vi "Inspect Certificate.vi"(11 "Certificate string":string) -> (3 "Certificates":T1(array[cluster]))   [LabVIEW 2013, in "Certification Authority.lvclass"]
uses:
  Certification Authority.lvclass
  <vilib>/LabVIEW Open Source Project/OpenSerializer.Base64/Base64_CharSet.vi
  <vilib>/Utility/error.llb/Error Cluster From Error Code.vi
  <vilib>/regexp/Match Regular Expression.xnode
  <vilib>/LabVIEW Open Source Project/OpenSerializer.Base64/Serializer.Base64.lvclass
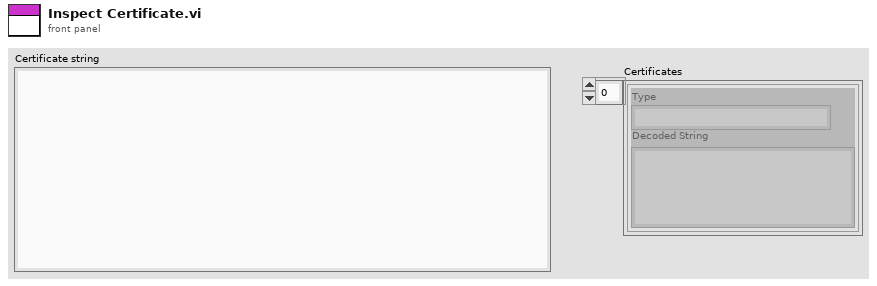
[diagram p1: front panel]
types:
  T1 = cluster{"Type":string, "Decoded String":string}[]
  T2 = cluster{"submatch 1":string, "spreadsheet string":string}
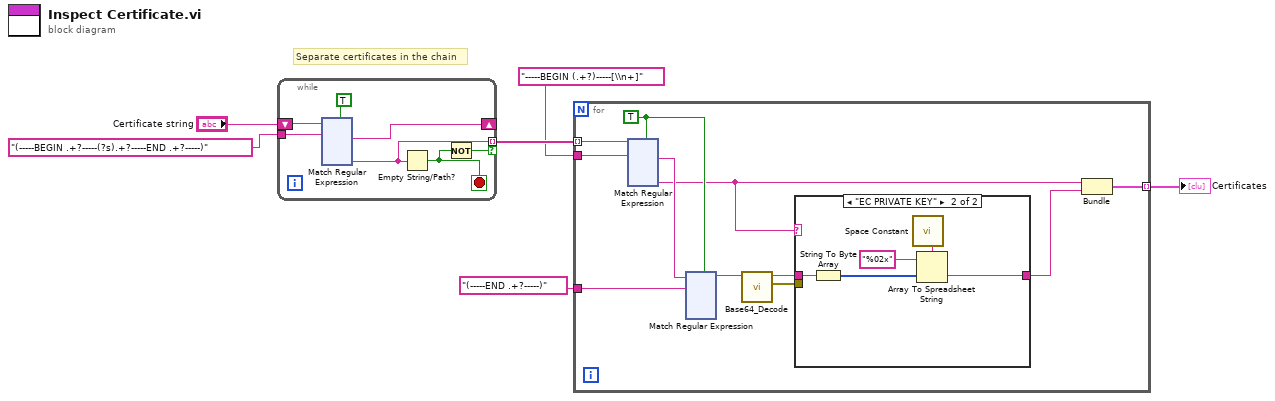
[diagram p0: block diagram]
diagram:
  # "Separate certificates in the chain"
  n1 = while {
    tunnel: "(-----BEGIN .+?-----(?s).+?-----END .+?-----)" ("regular expression") -> [w13]
    shift-right: [w11] -> _
    shift-left: "Certificate string" -> [w12]
    tunnel: [w9] -> w5 mode=indexing if=w8
    stop <- w7 stop-if-true
    n2 = xnode "Match Regular Expression"("input string"=w12, "regular expression"=w13, "multiline? (F)"=TRUE) -> ("after match"=w11:string, "submatch 1"=w9:string)  [unwired: 3 in, 4 out]
    n3 = Empty String/Path?(string/path=w9) -> (empty?=w7:bool)
    n4 = Not(x=w7) -> (.not. x?=w8:bool)
  }
  n5 = for {
    tunnel: w5 -> [w140] mode=indexing
    tunnel: "-----BEGIN (.+?)-----[\\n+]" ("regular expression") -> [w139]
    tunnel: "(-----END .+?-----)" ("regular expression") -> [w136]
    tunnel: [w134] -> w1 mode=indexing
    w137 = TRUE ("multiline? (F)")
    n6 = xnode "Match Regular Expression"("input string"=w140, "regular expression"=w139, "multiline? (F)"=w137) -> ("after match"=w138:string, "submatch 1"=w133:string)  [unwired: 3 in, 4 out]
    n7 = xnode "Match Regular Expression"("input string"=w138, "regular expression"=w136, "multiline? (F)"=w137) -> ("before match"=w135:string)  [unwired: 3 in, 5 out]
    n8 = call <vilib>:"Base64_Decode.vi"("Base64 String"=w135) -> ("error out"=w130:errorcluster, "Decoded String"=w132:string)  [unwired: 9 in]
    n9 = case shown="\"EC PRIVATE KEY\"" w133 {
      tunnel: w132 -> [w141 w146]
      tunnel: [w141 w145] -> w131
      tunnel: w130 -> [_ _]
      frame Default {
      }
      frame "EC PRIVATE KEY" {
        n10 = String To Byte Array(string=w146) -> (unsigned byte array=w144:u8[])
        n11 = call <vilib>:"Space Constant.vi"() -> ("String"=w142:string)
        n12 = Array To Spreadsheet String(delimiter (Tab)=w142, array=w144, 3:"%02x" ("format string")) -> (spreadsheet string=w145:string)
      }
    }
    n13 = Bundle("submatch 1"=w133, "spreadsheet string"=w131) -> (w134:T2)  [unwired: 1 in]
  }
  "Certificates" <- w1
